vi "Thorlabs_Shutter_ActiveX.vi"() -> ()   [LabVIEW 2023]
panel:
  in  "HWSerialNum":i32=68250849
  in  "error in (no error)":errorcluster caption="entrée d'erreur (pas d'erreur)"
  out "sortie d'erreur":errorcluster
  in  "stop":bool
  in  "MG17Motor":refnum<k7>(container)
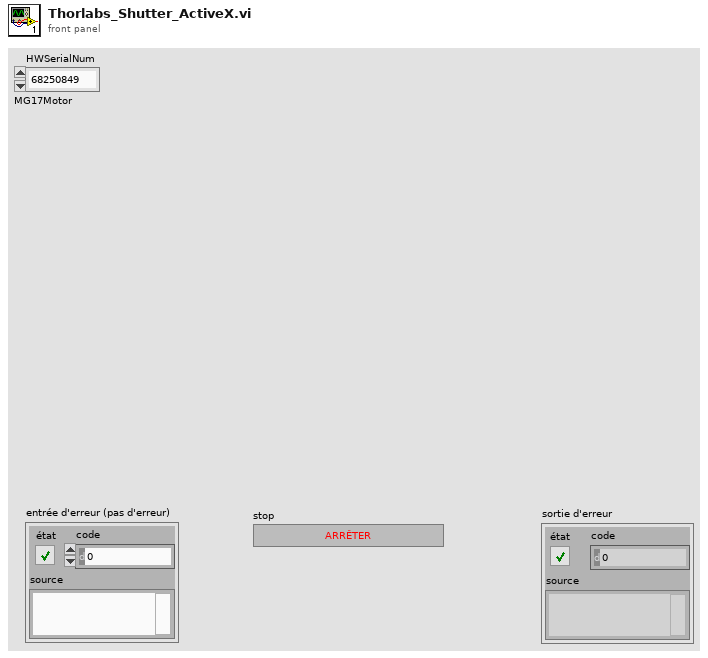
[diagram p1: front panel]
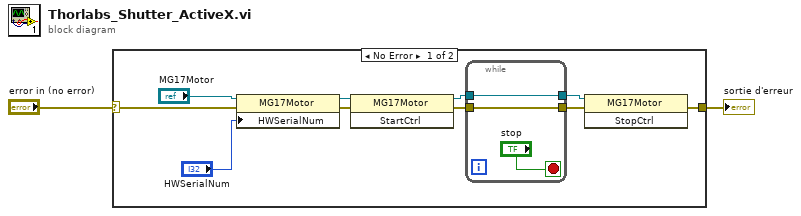
[diagram p0: block diagram]
diagram:
  n1 = case shown="No Error" "error in (no error)" {
    selector: "error in (no error)" -> [w3 w16]
    tunnel: [w4 w16] -> w2
    frame No Error {
      n2 = property on="Nœud de propriété" class="MG17Motor"(reference="MG17Motor", error in=w3, "HWSerialNum"="HWSerialNum") -> (reference out=w10:refnum<k7>, error out=w5:errorcluster)
      n3 = invoke on="Nœud de méthode" class="MG17Motor" method="StartCtrl"(reference=w10, error in=w5) -> (reference out=w9:refnum<k7>, error out=w6:errorcluster)  [unwired: 1 in, 1 out]
      n4 = while {
        tunnel: w9 -> [w14]
        tunnel: [w14] -> w8
        tunnel: [w13] -> w7
        tunnel: w6 -> [w13]
        stop <- "stop" stop-if-true
      }
      n5 = invoke on="Nœud de méthode" class="MG17Motor" method="StopCtrl"(reference=w8, error in=w7) -> (error out=w4:errorcluster)  [unwired: 1 in, 2 out]
    }
    frame Error {
    }
  }
  "sortie d'erreur" <- w2
